vi "Configure Measurement.vi"(6 "Manual Range (1000)":dbl=1000.0 format="%#.3f", 7 "Primary Function (0: DC Volts)":u16(ring) items=["DC Volts", "AC Volts", "AC+DC Volts", "DC Current", "AC Current", "AC+DC Current", "2-Wire Resistance", "Frequency", "Period", "Diode", "Continuity"], 8 "error in (no error)":errorcluster, 9 "Auto Range (T:Enable)":bool=TRUE, 10 "Secondary Function (1: AC Volts)":u16(ring)=1 items=["DC Volts", "AC Volts", "DC Current", "AC Current", "Frequency", "dB", "dBm"], 11 "VISA resource name":refnum<visa-resource-name>) -> (0 "error out":errorcluster, 3 "VISA resource name out":refnum<visa-resource-name>)   [LabVIEW 2020, in "BK Precision 5491B.lvlib"]
doc: "Configures the primary and secondary measurement type, resolution, and range on the instrument.\n\n<b>Note: When running this vi, secondary display will automatically be disabled. Use the Enable Secondary Display.vi</b> to enable it again.</b>"
uses:
  <instrlib>/BK Precision 5491B/BK Precision 5491B.lvlib
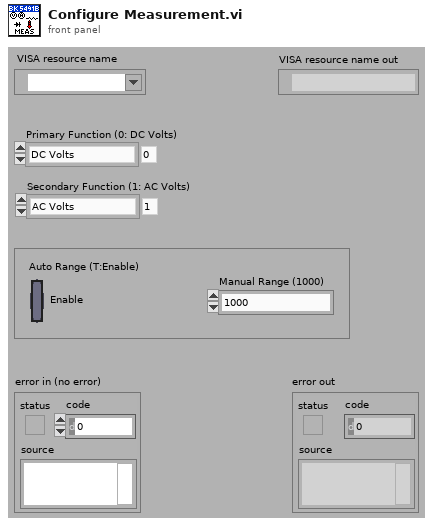
[diagram p1: front panel]
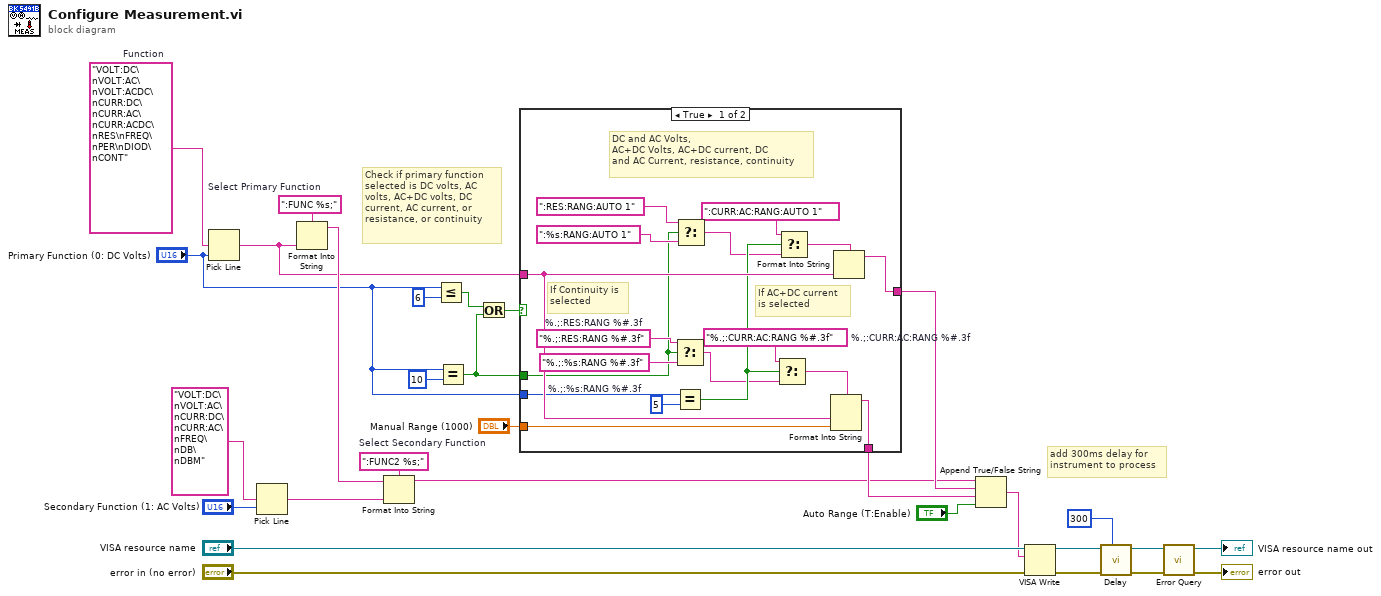
[diagram p0: block diagram]
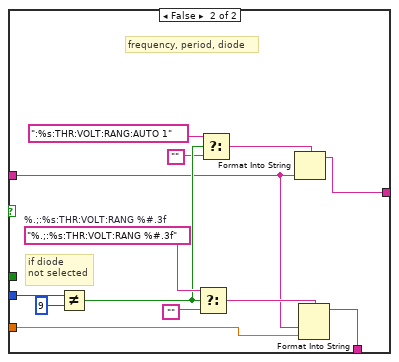
[diagram p2: hidden frame]
diagram:
  w20 = ":FUNC2 %s;"  # Select Secondary Function
  w24 = ":FUNC %s;"  # Select Primary Function
  w25 = "VOLT:DC\nVOLT:AC\nVOLT:ACDC\nCURR:DC\nCURR:AC\nCURR:ACDC\nRES\nFREQ\nPER\nDIOD\nCONT"  # Function
  # "add 300ms delay for\ninstrument to process"
  # "Check if primary function\nselected is DC volts, AC\nvolts, AC+DC volts, DC\ncurrent, AC current, or\nresistance, or continuity"
  n1 = Pick Line(multi-line string=w25, line index="Primary Function (0: DC Volts)") -> (output string=w17:string)  [unwired: 1 in]
  n2 = Pick Line(multi-line string="VOLT:DC\nVOLT:AC\nCURR:DC\nCURR:AC\nFREQ\nDB\nDBM", line index="Secondary Function (1: AC Volts)") -> (output string=w19:string)  [unwired: 1 in]
  n3 = Format Into String(format string=w24, w17) -> (resulting string=w18:string)  [unwired: 2 in, 1 out]
  n4 = Format Into String(format string=w20, initial string=w18, w19) -> (resulting string=w13:string)  [unwired: 1 in, 1 out]
  n5 = Less Or Equal?(x="Primary Function (0: DC Volts)", y=u16 6) -> (x <= y?=w9:bool)
  n6 = Equal?(x="Primary Function (0: DC Volts)", y=u16 10) -> (x = y?=w8:bool)
  n7 = Or(x=w9, y=w8) -> (x .or. y?=w10:bool)
  n8 = case shown="True" w10 {
    tunnel: w17 -> [w47 w50]
    tunnel: "Manual Range (1000)" -> [w46 w52]
    tunnel: [w45 w48] -> w16
    tunnel: [w44 w49] -> w15
    tunnel: w8 -> [w39 _]
    tunnel: "Primary Function (0: DC Volts)" -> [w37 w60]
    frame True {
      w32 = "%.;:CURR:AC:RANG %#.3f"  # %.;:CURR:AC:RANG %#.3f
      w41 = "%.;:RES:RANG %#.3f"  # %.;:RES:RANG %#.3f
      w43 = "%.;:%s:RANG %#.3f"  # %.;:%s:RANG %#.3f
      # "If AC+DC current\nis selected"
      # "If Continuity is\nselected"
      # "DC and AC Volts,\nAC+DC Volts, AC+DC current, DC\nand AC Current, resistance, continuity"
      n9 = Select(t=w41, s=w39, f=w43) -> (s? t:f=w35:string)
      n10 = Equal?(x=w37, y=u16 5) -> (x = y?=w36:bool)
      n11 = Select(t=":RES:RANG:AUTO 1", s=w39, f=":%s:RANG:AUTO 1") -> (s? t:f=w34:string)
      n12 = Select(t=w32, s=w36, f=w35) -> (s? t:f=w30:string)
      n13 = Select(t=":CURR:AC:RANG:AUTO 1", s=w36, f=w34) -> (s? t:f=w31:string)
      n14 = Format Into String(format string=w30, w47, w46) -> (resulting string=w44:string)  [unwired: 2 in, 1 out]
      n15 = Format Into String(format string=w31, w47) -> (resulting string=w45:string)  [unwired: 2 in, 1 out]
    }
    frame False {
      w58 = "%.;:%s:THR:VOLT:RANG %#.3f"  # %.;:%s:THR:VOLT:RANG %#.3f
      # "if diode\nnot selected"
      # "frequency, period, diode"
      n16 = Not Equal?(x=w60, y=u16 9) -> (x != y?=w56:bool)
      n17 = Select(t=w58, s=w56, f="") -> (s? t:f=w53:string)
      n18 = Select(t=":%s:THR:VOLT:RANG:AUTO 1", s=w56, f="") -> (s? t:f=w51:string)
      n19 = Format Into String(format string=w51, w50) -> (resulting string=w48:string)  [unwired: 2 in, 1 out]
      n20 = Format Into String(format string=w53, w50, w52) -> (resulting string=w49:string)  [unwired: 2 in, 1 out]
    }
  }
  n21 = Append True/False String(1:"Auto Range (T:Enable)", 2:w15, 3:w16, 4:w13) -> (0:w6:string)
  n22 = VISA Write(VISA resource name="VISA resource name", write buffer=w6, error in (no error)="error in (no error)") -> (VISA resource name out=w5:refnum<visa-resource-name>, error out=w2:errorcluster)  [unwired: 1 out]
  n23 = call <instrlib>:"Delay.vi"("Delay Time (0)"=u32 300, "error in (no error)"=w2, "VISA resource name"=w5) -> ("error out"=w3:errorcluster, "VISA resource name out"=w4:refnum<visa-resource-name>)  [unwired: 7 in]
  n24 = call <instrlib>:"Error Query.vi"("error in (no error)"=w3, "VISA resource name"=w4) -> ("error out"=→"error out":errorcluster, "VISA resource name out"=→"VISA resource name out":refnum<visa-resource-name>)  [unwired: 7 in, 1 out]
